vi "Get Camera Data.vi"(8 "error in (no error)":errorcluster, 11 "Camera in":refnum<class "Camera.lvclass">) -> (0 "error out":errorcluster, 1 "diameter (mm)":dbl, 2 "image":T1, 3 "Camera out":refnum<class "Camera.lvclass">, 5 "timestamp":timestamp)   [LabVIEW 2020, in "Camera.lvclass"]
uses:
  Camera.lvclass
  C:/Users/jharw/Documents/1 Folder to Rule them All/UMD/Inflation-Apparatus/src/Hardware/General Hardware.lvclass
  <vilib>/vision/Image Controls.llb/IMAQ Image.ctl
  General Hardware.lvclass/General Hardware.ctl
  Camera.lvclass/Camera.ctl
  General Hardware.lvclass
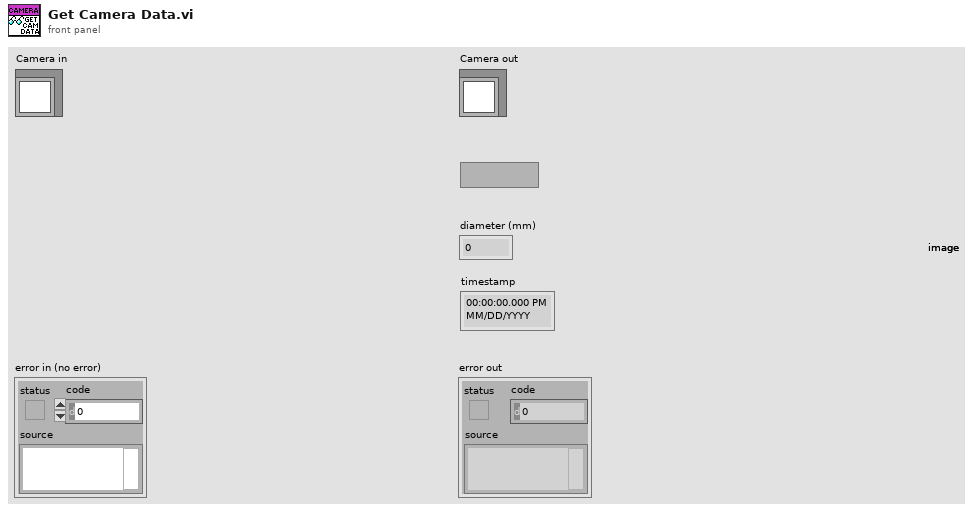
[diagram p1: front panel]
types:
  T1 = typedef "IMAQ Image.ctl" = refnum<image>
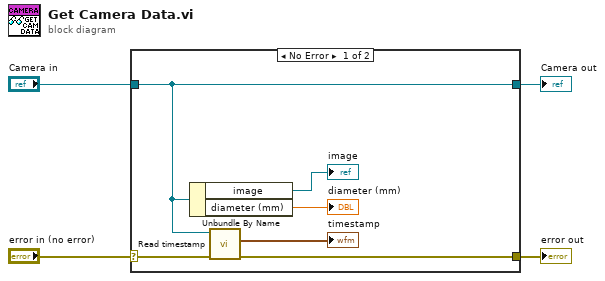
[diagram p0: block diagram]
diagram:
  n1 = case shown="No Error" "error in (no error)" {
    selector: "error in (no error)" -> [w6 w11]
    tunnel: [w5 w11] -> w3
    tunnel: [w8 w12] -> w1
    tunnel: "Camera in" -> [w8 w12]
    frame No Error {
      n2 = Unbundle By Name(w8) -> ("image"=→"image":T1, "diameter (mm)"=→"diameter (mm)":dbl)
      n3 = call "Read timestamp.vi"("error in (no error)"=w6, "General Hardware in"=w8) -> ("error out"=w5:errorcluster, "timestamp"=→"timestamp":timestamp)  [unwired: 7 in, 1 out]
    }
    frame Error {
    }
  }
  "error out" <- w3
  "Camera out" <- w1
